vi "SaveImages.vi"(0 "reference in":refnum<class "Control.lvclass">, 1 "Image path":path, 2 "Image URL":string, 5 "error in (no error)":errorcluster) -> (14 "reference out":refnum<class "Control.lvclass">, 15 "Image 1 URL":string, 16 "Image 2 URL":string, 19 "error out":errorcluster)   [LabVIEW 2014, in "Control.lvclass"]
uses:
  Control.lvclass
  Object_class/Object.lvclass
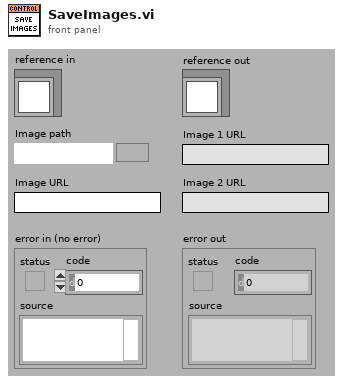
[diagram p1: front panel]
types:
  T1 = typedef "Object.lvclass/Attributes.ctl" = cluster{"UID":i32, "Type":string, "Coordinates":T2}
  T2 = typedef "Object.lvclass/Coordinates.ctl" = cluster{"Left":i32, "Top":i32, "Height":u32, "Width":u32}
  T3 = typedef "Control.lvclass/Attributes.ctl" = cluster{"Description":string, "Indicator":bool, "Default Value":variant, "Control Index":i32, "Label":refnum<class "Text.lvclass">, "Caption":refnum<class "Text.lvclass">, "Use Picture":bool, "Image 1":T4, "Image 2":T4}
  T4 = typedef "imagedata.ctl" = cluster{"image type":i32, "image depth":i32, "image":u8[], "mask":u8[], "colors":u32[], "Rectangle":cluster{"left":i16, "top":i16, "right":i16, "bottom":i16}}
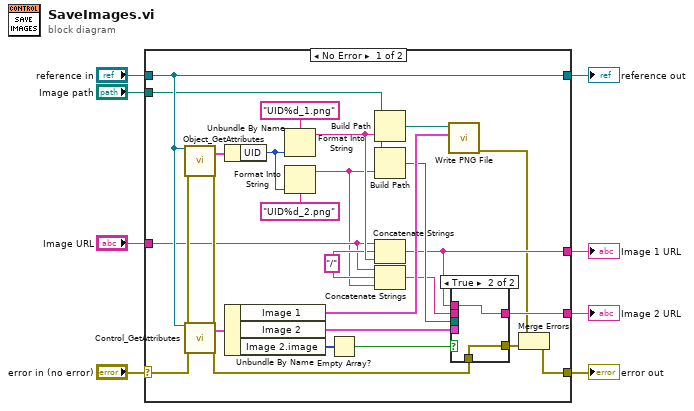
[diagram p0: block diagram]
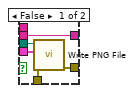
[diagram p2: hidden frame]
diagram:
  n1 = case shown="No Error" "error in (no error)" {
    selector: "error in (no error)" -> [w32 w43]
    tunnel: [w9 w43] -> w7
    tunnel: [w33 w42] -> w5
    tunnel: "reference in" -> [w33 w42]
    tunnel: "Image path" -> [w23 _]
    tunnel: "Image URL" -> [w17 _]
    tunnel: [w13 _] -> w2
    tunnel: [w14 _] -> w1
    frame No Error {
      w18 = "/"
      n2 = call "Object_GetAttributes.vi"("reference in"=w33, "error in (no error)"=w32) -> ("Data"=w31:T1, "error out"=w20:errorcluster)  [unwired: 14 in, 2 out]
      n3 = call "Control_GetAttributes.vi"("reference in"=w33, "error in (no error)"=w20) -> ("Data"=w34:T3, "error out"=w10:errorcluster)  [unwired: 14 in, 2 out]
      n4 = Unbundle By Name(w31) -> ("UID"=w24:i32)
      n5 = Unbundle By Name(w34) -> ("Image 1"=w29:T4, "Image 2"=w26:T4, "Image 2.image"=w28:u8[])
      n6 = Format Into String(format string="UID%d_1.png", w24) -> (resulting string=w19:string)  [unwired: 2 in, 1 out]
      n7 = Format Into String(format string="UID%d_2.png", w24) -> (resulting string=w16:string)  [unwired: 2 in, 1 out]
      n8 = Empty Array?(array=w28) -> (empty?=w27:bool)
      n9 = Build Path(base path=w23, name or relative path=w19) -> (appended path=w21:path)
      n10 = Build Path(base path=w23, name or relative path=w16) -> (appended path=w22:path)
      n11 = Concatenate Strings(w17, w18, w19) -> (w13:string)
      n12 = Concatenate Strings(w17, w18, w16) -> (w15:string)
      n13 = call <vilib>:"Write PNG File.vi"("image data"=w29, "path to PNG file"=w21) -> ("error out"=w11:errorcluster)  [unwired: 8 in, 1 out]
      n14 = case shown="True" w27 {
        tunnel: w26 -> [w39 _]
        tunnel: w22 -> [w38 _]
        tunnel: [w37 w41] -> w14
        tunnel: w15 -> [w37 _]
        tunnel: w13 -> [_ w41]
        tunnel: w10 -> [w36 w40]
        tunnel: [w35 w40] -> w12
        frame False {
          n15 = call <vilib>:"Write PNG File.vi"("error in (no error)"=w36, "image data"=w39, "path to PNG file"=w38) -> ("error out"=w35:errorcluster)  [unwired: 7 in, 1 out]
        }
        frame True {
        }
      }
      n16 = Merge Errors(w11, w12) -> (w9:errorcluster)
    }
    frame Error {
    }
  }
  "error out" <- w7
  "reference out" <- w5
  "Image 1 URL" <- w2
  "Image 2 URL" <- w1
